vi "Set DDG Address.vi"(6 "address":u8, 7 "t3":u8, 9 "t2":u8, 10 "t1":u8, 11 "t0":u8) -> (3 "function return":u32)   [LabVIEW 2018, in "AndorSDK.lvlib"]
doc: "EXPNETTYPE unsigned int WINAPI SetDDGAddress(BYTE t0, BYTE t1, BYTE t2, BYTE t3, BYTE address);"
uses:
  AndorSDK.lvlib
  ATMCD32D.dll
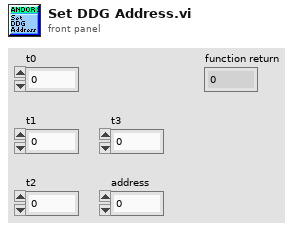
[diagram p1: front panel]
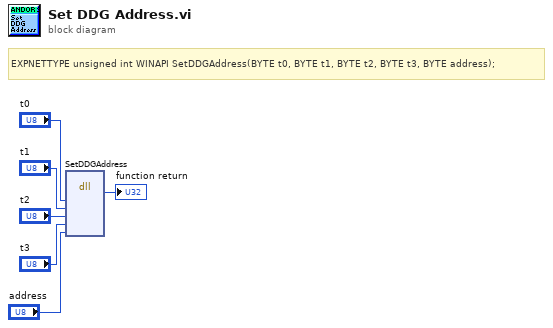
[diagram p0: block diagram]
diagram:
  # "EXPNETTYPE unsigned int WINAPI SetDDGAddress(BYTE t0, BYTE t1, BYTE t2, BYTE t3, BYTE address);"
  n1 = dll-call lib="PTH2babs E\nPersönliches02 - Arbeit03-HiwijobsLabviewCodelibANDOR\tAndor SDK\nATMCD32D.*" fn="SetDDGAddress"("t0"="t0", "t1"="t1", "t2"="t2", "t3"="t3", "address"="address") -> (→"function return":u32)  [unwired: 8 in, 2 out]
